vi "Close Hardware.vi"(8 "error in (no error)":errorcluster, 11 "Inst.SPC in":refnum<class "Inst.SPC.lvclass">) -> (0 "error out":errorcluster, 3 "Inst.SPC out":refnum<class "Inst.SPC.lvclass">)   [LabVIEW 2019, in "Inst.SPC.lvclass"]
uses:
  Inst.SPC.lvclass
  Inst.SPC.lvclass/Inst.SPC.ctl
  <userlib>/LevyLab/Instrument Framework/Instrument Types/VSource/Instrument.VSource.lvclass
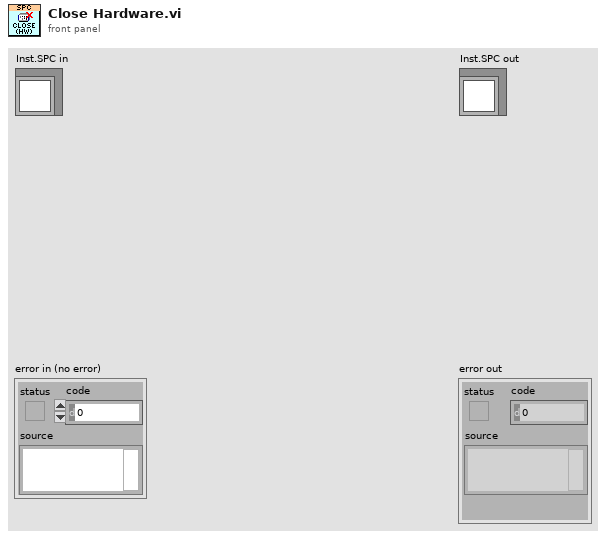
[diagram p1: front panel]
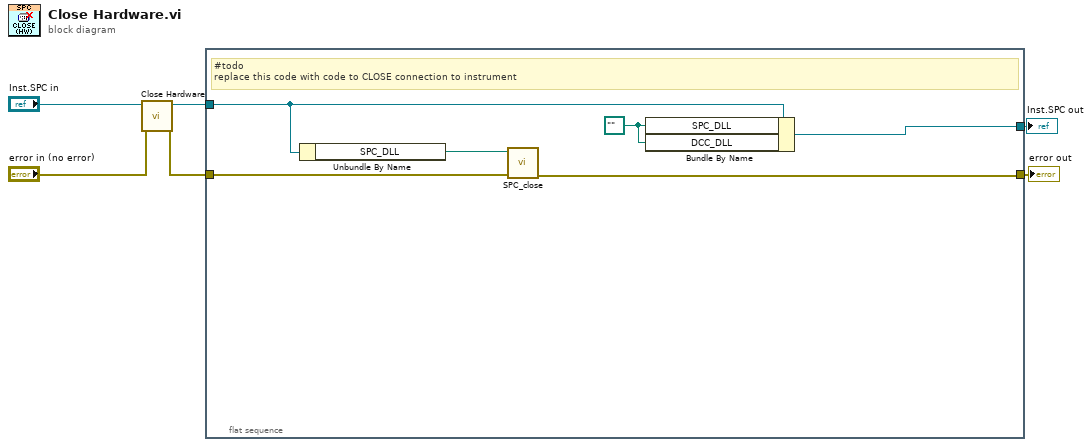
[diagram p0: block diagram]
diagram:
  n1 = call-parent "Close Hardware.vi"("error in (no error)"="error in (no error)", "Instrument in"="Inst.SPC in") -> ("error out"=w4:errorcluster, "Instrument out"=w2:refnum<class "Inst.SPC.lvclass">)  [unwired: 8 in]
  n2 = flat-sequence {
    tunnel: w4 -> [w12]
    tunnel: [w11] -> w3
    tunnel: w2 -> [w10]
    tunnel: [w9] -> w1
    frame #0 {
      w7 = path "" ("Configuration.SPC_DLL")
      # "#todo\nreplace this code with code to CLOSE connection to instrument"
      n3 = Unbundle By Name(w10) -> ("SPC_DLL"=w8:path)
      n4 = call "SPC_close.vi"("Error In"=w12, "DLL Path"=w8) -> ("Error Out"=w11:errorcluster)  [unwired: 8 in, 1 out]
      n5 = Bundle By Name(cluster=w10, "SPC_DLL"=w7, "DCC_DLL"=w7) -> (w9:refnum<class "Inst.SPC.lvclass">)
    }
  }
  "error out" <- w3
  "Inst.SPC out" <- w1
